vi "Main - Search VI Ref (SubVI).vi"(8 "Error In":errorcluster, 10 "VI Name to Search":string, 11 "VI Refs":refnum<vi>[](array[refnum])) -> (0 "Error Out":errorcluster, 1 "VI Ref Found":refnum<vi>, 3 "Found?":bool)   [LabVIEW 2019]
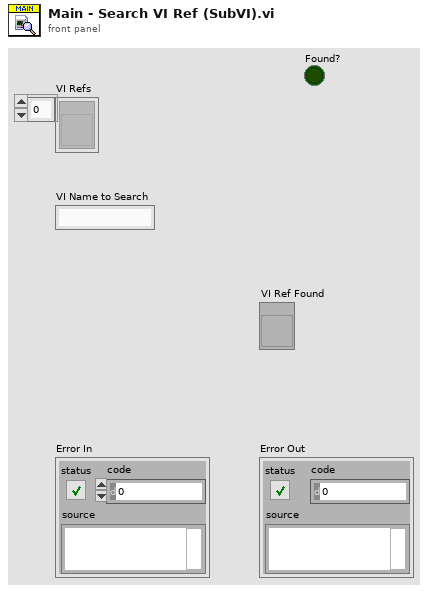
[diagram p1: front panel]
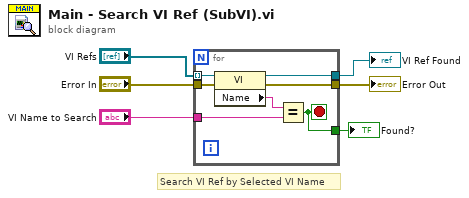
[diagram p0: block diagram]
diagram:
  # "Search VI Ref by Selected VI Name"
  n1 = for {
    tunnel: "Error In" -> [w13]
    tunnel: [w12] -> w6
    tunnel: "VI Refs" -> [w11] mode=indexing
    tunnel: "VI Name to Search" -> [w9]
    tunnel: [w8] -> w4
    tunnel: [w7] -> w1
    stop <- w7 stop-if-true
    n2 = property class="VI"(reference=w11, error in=w13) -> (reference out=w8:refnum<vi>, error out=w12:errorcluster, "Name"=w10:string)
    n3 = Equal?(x=w10, y=w9) -> (x = y?=w7:bool)
  }
  "Error Out" <- w6
  "VI Ref Found" <- w4
  "Found?" <- w1
